vi "CSDB_Transfer.FindFreeID.vi"(3 "error in (no error)":errorcluster, 4 "table":string, 5 "# of IDs":dbl=1.0, 6 "connection reference":T1) -> (0 "error out":errorcluster, 1 "FreeIDs":i32[](array[numeric]), 2 "connection reference out":T1)   [LabVIEW 2014, in "CSDB_Transfer.lvlib"]
uses:
  CSDB_Transfer.lvlib
  <vilib>/addons/database/Connection.llb/Conn ObjectReference.ctl
  CSDB_Common/CSDB_Common.lvlib
  <vilib>/addons/database/NI_Database_API.lvlib
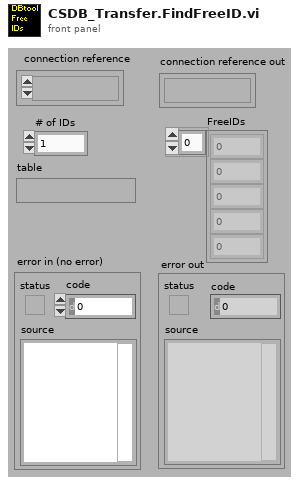
[diagram p1: front panel]
types:
  T1 = typedef "NI_Database_API.lvlib/Conn ObjectReference.ctl" = refnum<k1>
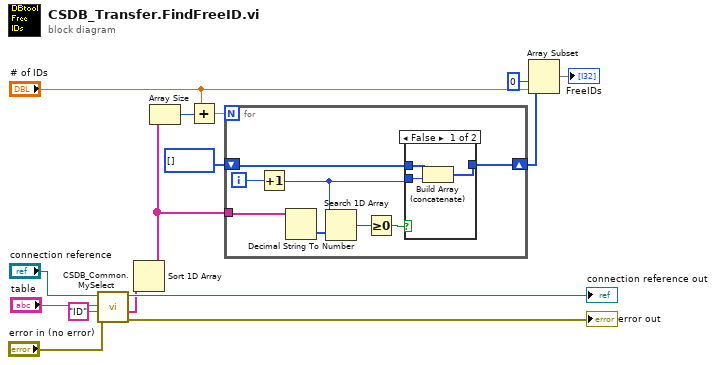
[diagram p0: block diagram]
diagram:
  n1 = call "CSDB_Common.MySelect.vi"("error in (no error)"="error in (no error)", "column"="ID", "table"="table", "connection reference"="connection reference") -> ("error out"=→"error out":errorcluster, "1d output array"=w11:string[], "connection reference out"=→"connection reference out":T1)  [unwired: 3 in]
  n2 = Sort 1D Array(array=w11) -> (sorted array=w10:string[])
  n3 = Array Size(array=w10) -> (size(s)=w5:i32)
  n4 = Add(x="# of IDs", y=w5) -> (x+y=w4:dbl)
  n5 = for {
    N: w4 -> [_]
    tunnel: w10 -> [w23]
    shift-right: [w17] -> w8
    shift-left: i32[] [] -> [w16]
    i -> [w22]
    n6 = Increment(x=w22) -> (x+1=w18:i32)
    n7 = Decimal String To Number(string=w23) -> (number=w19:i32[])  [unwired: 2 in, 1 out]
    n8 = Search 1D Array(1D array=w19, element=w18) -> (index of element=w21:i32)  [unwired: 1 in]
    n9 = Greater Or Equal To 0?(x=w21) -> (x >= 0?=w20:bool)
    n10 = case shown="False" w20 {
      tunnel: w18 -> [w25 _]
      tunnel: [w24 w27] -> w17
      tunnel: w16 -> [w26 w27]
      frame False {
        n11 = Build Array (concatenate)(w26, w25) -> (w24:i32[])
      }
      frame True {
      }
    }
  }
  n12 = Array Subset(array=w8, index=0, length="# of IDs") -> (→"FreeIDs":i32[])
